vi "Digital Ramp Pattern Generator.vi"(0 "Number of Digital Lines":u32, 5 "Number of Samples":u32, 11 "error in":errorcluster) -> (4 "Port Digital Data":u32[](array[numeric]), 15 "error out":errorcluster)   [LabVIEW 2019]
doc: "<B>Digital Ramp Pattern Generator</B> generates Ramp based Digital Output Data couting from 0 upto (2^N)-1 where \"N\" represents the Number of Digital Lines. The Ramp based pattern is given out as 1D array of U32 Port Digital Data."
panel:
  # "Outputs"
  # "Inputs"
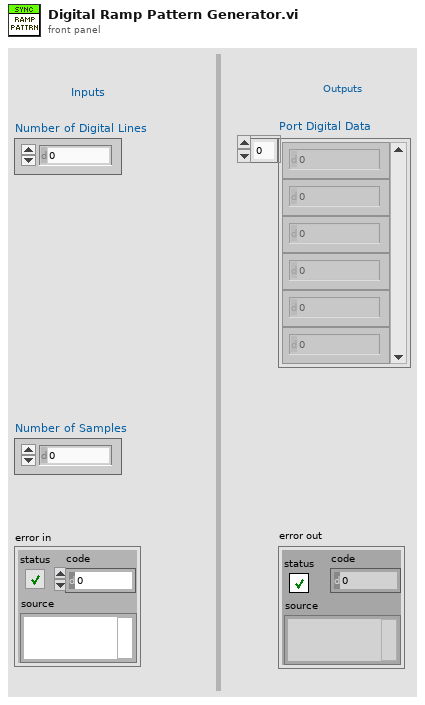
[diagram p1: front panel]
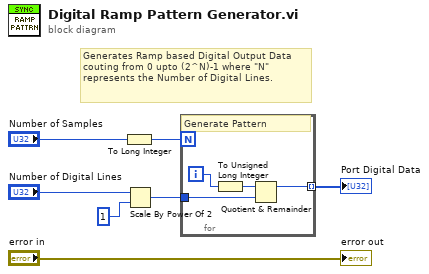
[diagram p0: block diagram]
diagram:
  # "Generates Ramp based Digital Output Data couting from 0 upto (2^N)-1 where \"N\" represents the Number of Digital Lines."
  n1 = To Long Integer(number="Number of Samples") -> (32bit integer=w6:i32)
  n2 = Scale By Power Of 2(n="Number of Digital Lines", x=u32 1) -> (x*2^n=w3:u32)
  n3 = for {
    N: w6 -> [_]
    tunnel: w3 -> [w11]
    tunnel: [w9] -> w5 mode=indexing
    i -> [w10]
    # "Generate Pattern"
    n4 = To Unsigned Long Integer(number=w10) -> (unsigned 32bit integer=w8:u32)
    n5 = Quotient & Remainder(x=w8, y=w11) -> (x-y*floor(x/y)=w9:u32)  [unwired: 1 out]
  }
  "Port Digital Data" <- w5
  "error out" <- "error in"
